vi "Add(DBL).vi"(8 "错误输入":errorcluster, 10 "Value":dbl, 11 "TagName":string) -> (0 "错误输出":errorcluster)   [LabVIEW 2013, in "Tag Data by Variant.lvlib"]
uses:
  Tag Data by Variant.lvlib
  Custom def/mode.ctl
  Core/TagVar Data(DBL).vi
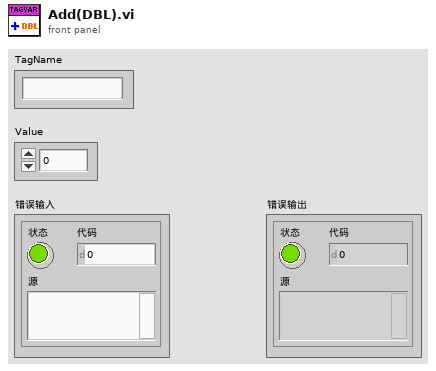
[diagram p1: front panel]
types:
  T1 = typedef "Tag Data by Variant.lvlib/mode.ctl" = enum16{"初始化", "加入", "删除", "读取", "读取所有", "清除"}
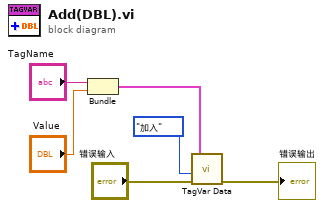
[diagram p0: block diagram]
diagram:
  n1 = Bundle("TagName"="TagName", "Value"="Value") -> (w1:cluster{"TagName":string, "Value":dbl})  [unwired: 1 in]
  n2 = call-poly "TagVar Data.vi"("错误输入"="错误输入", "method"=mode."加入", "TagData In"=w1) -> ("错误输出"=→"错误输出":errorcluster)  [unwired: 6 in, 2 out]
